vi "TestExec.Result, File Data Objs.vi"(7 "Module Q Name":string, 8 "error in":errorcluster, 10 "File Data Objs":T1[](array[typedef]), 11 "Q In":refnum<queue>) -> (0 "error out":errorcluster)   [LabVIEW 2024]
uses:
  <vilib>/KATE/Queues/Q.Element.ctl
  Reports/Report.Result FileDataObject.ctl
  <vilib>/KATE/Queues/Queue Utils.lvlib
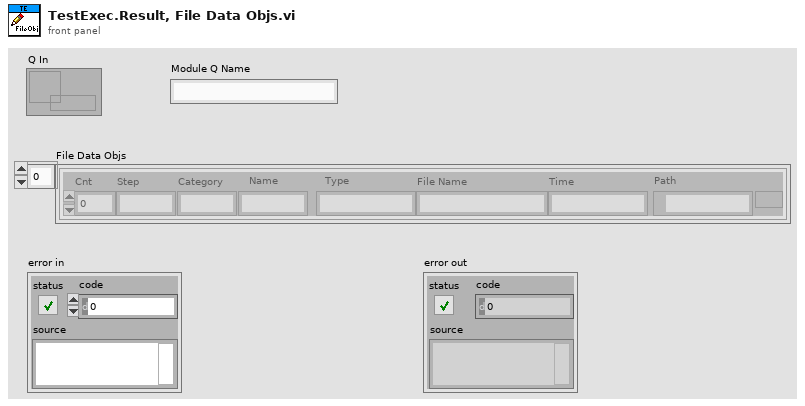
[diagram p1: front panel]
types:
  T1 = typedef "Report.Result FileDataObject.ctl" = cluster{"Cnt":i32, "Step":string, "Category":string, "Name":string, "Type":string, "File Name":string, "Time":string, "Path":path}
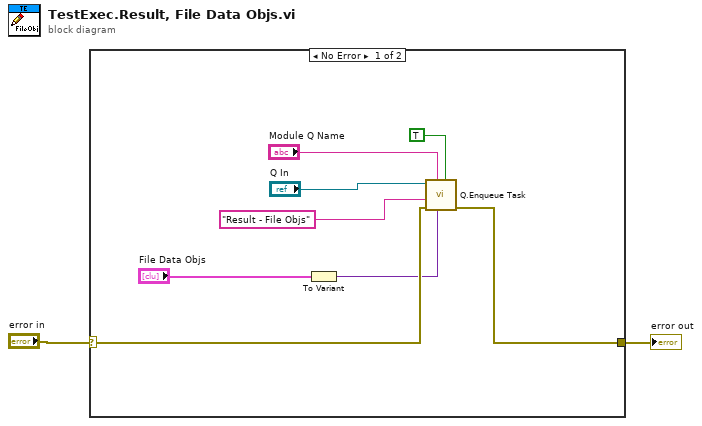
[diagram p0: block diagram]
diagram:
  n1 = case shown="No Error" "error in" {
    selector: "error in" -> [w7 w11]
    tunnel: [w8 w11] -> w1
    frame No Error {
      n2 = To Variant(anything="File Data Objs") -> (Variant=w6:variant)
      n3 = call <vilib>:"Q.Enqueue Task.vi"("Top of Q"=TRUE, "Data1"=w6, "Q Name"="Module Q Name", "Error In"=w7, "Task Name"="Result - File Objs" ("Cmd"), "Q In"="Q In") -> ("error out"=w8:errorcluster)  [unwired: 4 in, 1 out]
    }
    frame Error {
    }
  }
  "error out" <- w1
